vi "Get Next String Token.vi"(8 "error in (no error)":errorcluster, 9 "Final":bool, 10 "inputString":string, 11 "TEI9150 in":refnum<class "Tovey 9150.lvclass">) -> (0 "error out":errorcluster, 1 "remainingString":string, 2 "extractedSegment":string, 3 "TEI9150 out":refnum<class "Tovey 9150.lvclass">)   [LabVIEW 2015, in "Tovey 9150.lvclass"]
uses:
  Tovey 9150.lvclass
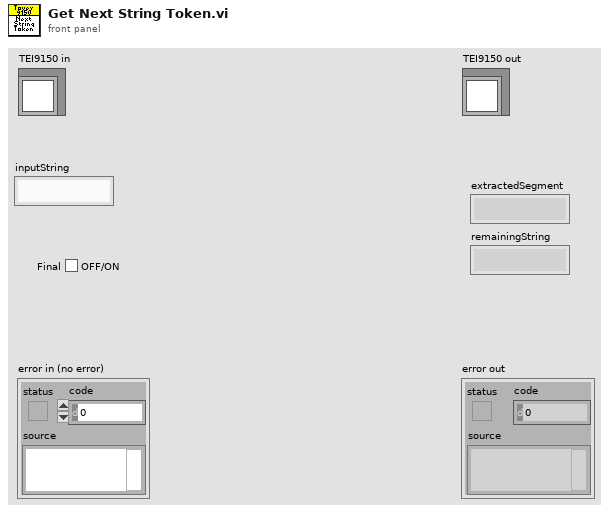
[diagram p1: front panel]
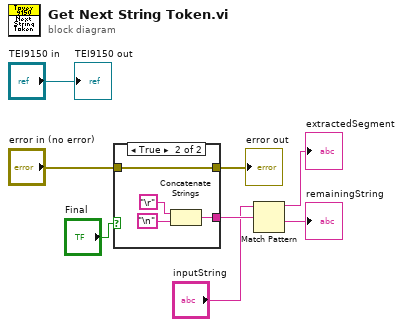
[diagram p0: block diagram]
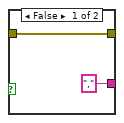
[diagram p2: hidden frame]
diagram:
  n1 = case shown="True" "Final" {
    tunnel: ["," w12] -> w7
    tunnel: "error in (no error)" -> [w10 w11]
    tunnel: [w10 w11] -> w2
    frame False {
    }
    frame True {
      n2 = Concatenate Strings("\r", "\n") -> (w12:string)
    }
  }
  "error out" <- w2
  n3 = Match Pattern(string="inputString", regular expression=w7) -> (before substring=→"extractedSegment":string, after substring=→"remainingString":string)  [unwired: 1 in, 2 out]
  "TEI9150 out" <- "TEI9150 in"
